vi "RP generate pulse pattern.vi"(9 "Waveform parameters":T1={"Start magnitude"=1000.0, "Magnitude increment"=1000.0, "Number of pulses"=8, "Ramp length"=32, "Top  length"=480, "Threshold "=3000, "Processing delay"=480, "Stop after"=1, "Detector window"=480, "Upper limit"=8191, "Lower limit"=-8192} {"Lower limit" format="%d (0x%x)"; "Upper limit" format="%d (0x%x)"; "Detector window" format="%dpts"; "Stop after" format="%d sweep(s)"}, 11 "Baseline start":u16=128) -> (1 "Step length":u32=2048, 2 "Waveform length":u32, 3 "Waveform":i16[](array[numeric]), 5 "Waveform Graph":dbl[](graph))   [LabVIEW 2024]
uses:
  Waform generation/Waveform parameters.ctl
panel:
  in  "# Steps":i32
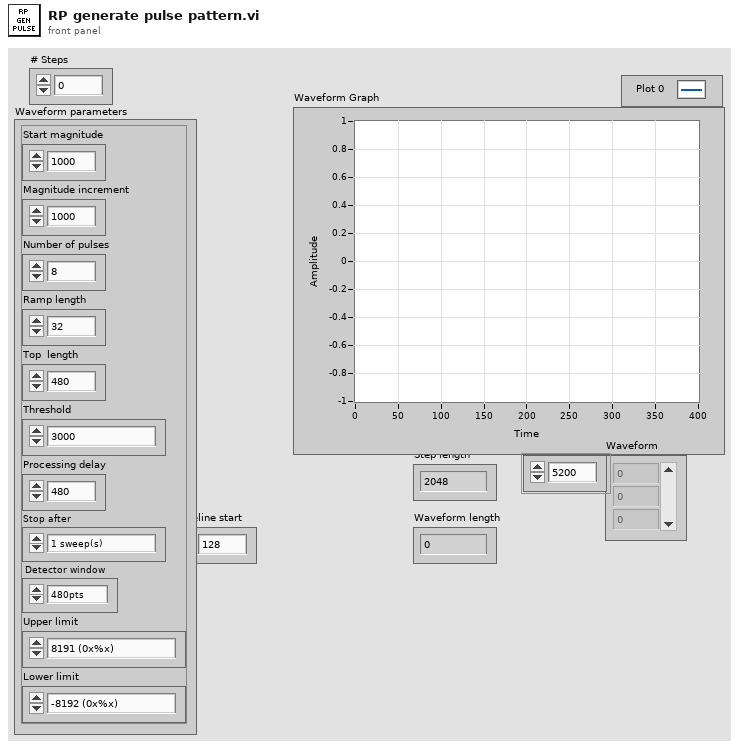
[diagram p1: front panel]
types:
  T1 = typedef "Waveform parameters.ctl" = cluster{"Start magnitude":dbl, "Magnitude increment":dbl, "Number of pulses":i32, "Ramp length":i32, "Top  length":i32, "Threshold ":i32, "Processing delay":u16, "Stop after":u16, "Detector window":i32, "Upper limit":i16, "Lower limit":i16}
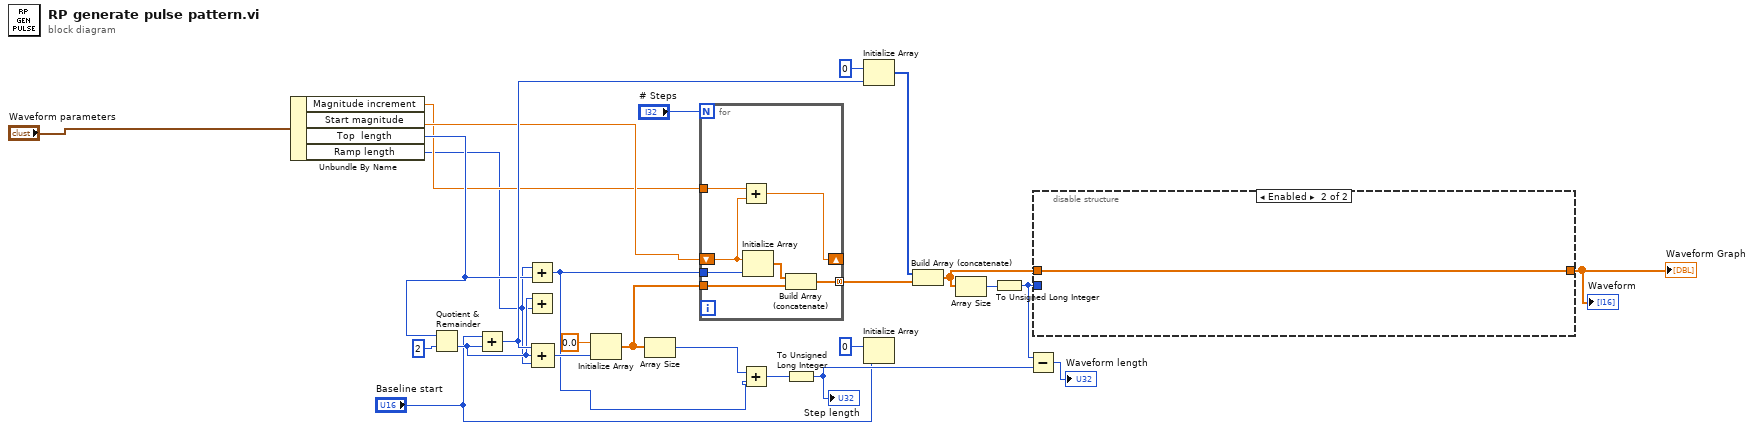
[diagram p0: block diagram]
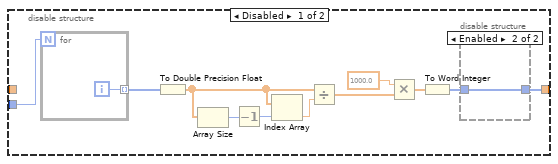
[diagram p2: hidden frame]
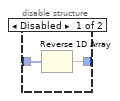
[diagram p3: hidden frame]
diagram:
  n1 = Unbundle By Name("Waveform parameters") -> ("Magnitude increment"=w2:dbl, "Start magnitude"=w3:dbl, "Top  length"=w4:i32, "Ramp length"=w1:i32)
  n2 = Quotient & Remainder(x=w4, y=u16 2) -> (floor(x/y)=w19:i32)  [unwired: 1 out]
  n3 = Add(x="Baseline start", y=w19) -> (x+y=w23:i32)
  n4 = Add(x=w1, y=w4) -> (x+y=w7:i32)
  n5 = Add(x=w19, y=w1) -> ()  [unwired: 1 out]
  n6 = Compound Arithmetic op=ADD(w23, w19, w1) -> (w22:i32)
  n7 = Initialize Array(0.0 ("element"), w22) -> (w9:dbl[])
  n8 = Array Size(array=w9) -> (size(s)=w16:i32)
  n9 = for {
    N: "# Steps" -> [_]
    tunnel: w7 -> [w33]
    tunnel: w9 -> [w31]
    tunnel: [w30] -> w8 mode=concatenating
    tunnel: w2 -> [w28]
    shift-right: [w27] -> _
    shift-left: w3 -> [w29]
    n10 = Add(x=w28, y=w29) -> (x+y=w27:dbl)
    n11 = Initialize Array(w29, w33) -> (w32:dbl[])
    n12 = Build Array (concatenate)(w32, w31) -> (w30:dbl[])
  }
  n13 = Add(x=w16, y=w7) -> (x+y=w17:i32)
  n14 = To Unsigned Long Integer(number=w17) -> (unsigned 32bit integer=w15:u32)
  "Step length" <- w15
  n15 = Initialize Array(i16 0, w23) -> (w24:i16[])
  n16 = Initialize Array(i16 0, "Baseline start") -> ()  [unwired: 1 out]
  n17 = Build Array (concatenate)(w24, w8) -> (w11:dbl[])
  n18 = Array Size(array=w11) -> (size(s)=w18:i32)
  n19 = To Unsigned Long Integer(number=w18) -> (unsigned 32bit integer=w13:u32)
  n20 = Subtract(x=w13, y=w15) -> (x-y=→"Waveform length":u32)
  n21 = disable-structure shown="Enabled" {
    disable-tunnel: w13 -> [w44 _]
    disable-tunnel: [w34 w49] -> w12
    disable-tunnel: w11 -> [_ w49]
    frame Disabled {
      n22 = for {
        N: w44 -> [_]
        tunnel: [w48] -> w43 mode=indexing
        i -> [w48]
      }
      n23 = To Double Precision Float(number=w43) -> (double precision float=w39:dbl[])
      n24 = Array Size(array=w39) -> (size(s)=w42:i32)
      n25 = Decrement(x=w42) -> (x-1=w41:i32)
      n26 = Index Array(array=w39, index=w41) -> (element=w40:dbl)
      n27 = Divide(x=w39, y=w40) -> (x/y=w38:dbl[])
      n28 = Multiply(x=1000.0, y=w38) -> (x*y=w36:dbl[])
      n29 = To Word Integer(number=w36) -> (16bit integer=w35:i16[])
      n30 = disable-structure shown="Enabled" {
        disable-tunnel: w35 -> [w46 w47]
        disable-tunnel: [w45 w47] -> w34
        frame Disabled {
          n31 = Reverse 1D Array(array=w46) -> (reversed array=w45:i16[])
        }
        frame Enabled {
        }
      }
    }
    frame Enabled {
    }
  }
  "Waveform Graph" <- w12
  "Waveform" <- w12
